vi "NaN_screening.vi"(11 "Input":T1 {"File Location" items=["Currently Writing"=-3, "Labview Files"=-2, "Mars Data Processing Factility"=-1, "Local Cache "=0, "Old Storage"=1, "Storage"=2]; "Estimate Source" items=["Any Source."=-2, "No Shot"=-1, "Basic Labview Estimate"=0, "IDL Estimate From Andrew"=1, "IDL Estimate From Keith"=2, "Old Metadata"=3]}) -> (3 "Output":T1 {"File Location" items=["Currently Writing"=-3, "Labview Files"=-2, "Mars Data Processing Factility"=-1, "Local Cache "=0, "Old Storage"=1, "Storage"=2]; "Estimate Source" items=["Any Source."=-2, "No Shot"=-1, "Basic Labview Estimate"=0, "IDL Estimate From Andrew"=1, "IDL Estimate From Keith"=2, "Old Metadata"=3]})   [LabVIEW 2012]
uses:
  Public API/Post_Dust_Event.ctl
  Estimate_source.ctl
  File_location.ctl
panel:
  # "Dust Event"
  # "Dust Event"
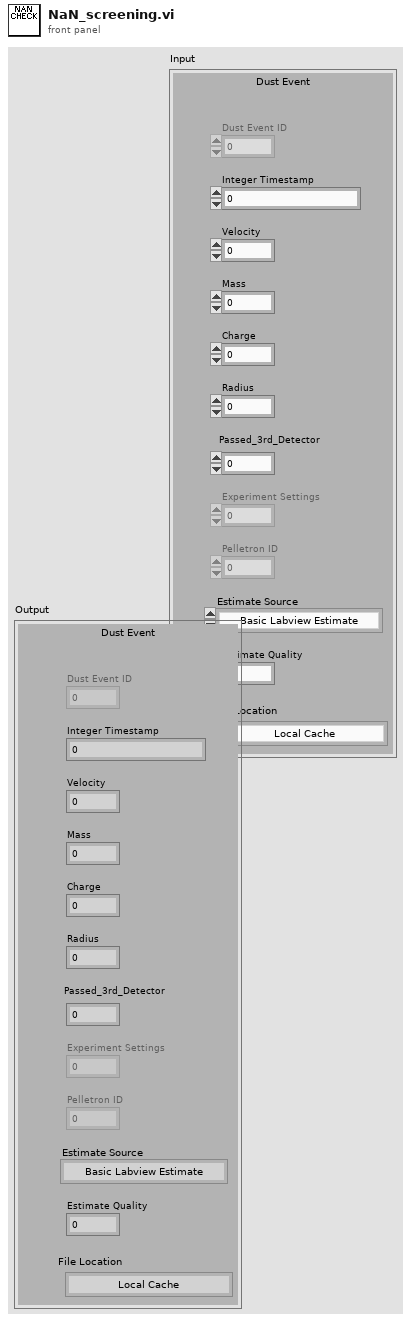
[diagram p1: front panel]
types:
  T1 = typedef "Post_Dust_Event.ctl" = cluster{"Dust Event ID":i64, "Integer Timestamp":i64, "Velocity":sgl, "Mass":sgl, "Charge":sgl, "Radius":sgl, "Passed_3rd_Detector":i8, "Experiment Settings":dbl, "Pelletron ID":i32, "Estimate Source":T2, "Estimate Quality":sgl, "File Location":T3, "id_dust_info":dbl}
  T2 = typedef "Estimate_source.ctl" = i8
  T3 = typedef "File_location.ctl" = i8
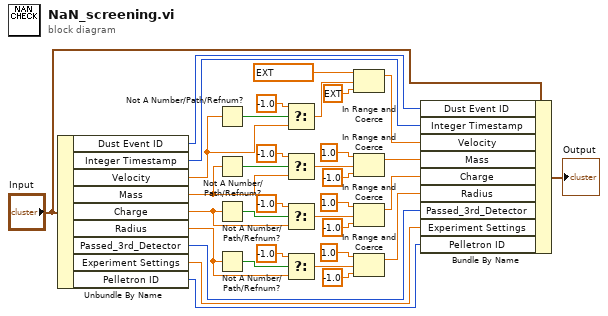
[diagram p0: block diagram]
diagram:
  n1 = Unbundle By Name("Input") -> ("Dust Event ID"=w33:i64, "Integer Timestamp"=w32:i64, "Velocity"=w19:sgl, "Mass"=w21:sgl, "Charge"=w23:sgl, "Radius"=w18:sgl, "Passed_3rd_Detector"=w31:i8, "Experiment Settings"=w30:dbl, "Pelletron ID"=w29:i32)
  n2 = Not A Number/Path/Refnum?(number/path/refnum=w19) -> (NaN/Path/Refnum?=w20:bool)
  n3 = Not A Number/Path/Refnum?(number/path/refnum=w21) -> (NaN/Path/Refnum?=w22:bool)
  n4 = Not A Number/Path/Refnum?(number/path/refnum=w23) -> (NaN/Path/Refnum?=w25:bool)
  n5 = Not A Number/Path/Refnum?(number/path/refnum=w18) -> (NaN/Path/Refnum?=w17:bool)
  n6 = Select(t=-1.0 ("y"), s=w20, f=w19) -> (s? t:f=w14:dbl)
  n7 = Select(t=-1.0 ("y"), s=w22, f=w21) -> (s? t:f=w10:dbl)
  n8 = Select(t=-1.0 ("y"), s=w25, f=w23) -> (s? t:f=w4:dbl)
  n9 = Select(t=-1.0 ("y"), s=w17, f=w18) -> (s? t:f=w2:dbl)
  n10 = In Range and Coerce(upper limit=ext 299792458.0, x=w14, lower limit=ext -1.0) -> (coerced(x)=w13:ext)  [unwired: 1 out]
  n11 = In Range and Coerce(upper limit=1.0, x=w10, lower limit=-1.0) -> (coerced(x)=w9:dbl)  [unwired: 1 out]
  n12 = In Range and Coerce(upper limit=1.0, x=w4, lower limit=-1.0) -> (coerced(x)=w3:dbl)  [unwired: 1 out]
  n13 = In Range and Coerce(upper limit=1.0, x=w2, lower limit=-1.0) -> (coerced(x)=w1:dbl)  [unwired: 1 out]
  n14 = Bundle By Name(cluster="Input", "Dust Event ID"=w33, "Integer Timestamp"=w32, "Velocity"=w13, "Mass"=w9, "Charge"=w3, "Radius"=w1, "Passed_3rd_Detector"=w31, "Experiment Settings"=w30, "Pelletron ID"=w29) -> (→"Output":T1)
